vi "Is Last Run.vi"(8 "error in (no error)":errorcluster, 10 "Last Run?":bool, 11 "Model in":refnum<class "Model.lvclass">) -> (0 "error out":errorcluster, 2 "Stop":bool, 3 "Model out":refnum<class "Model.lvclass">)   [LabVIEW 2016, in "Model.lvclass"]
uses:
  Model.lvclass
  Model.lvclass/Model.ctl
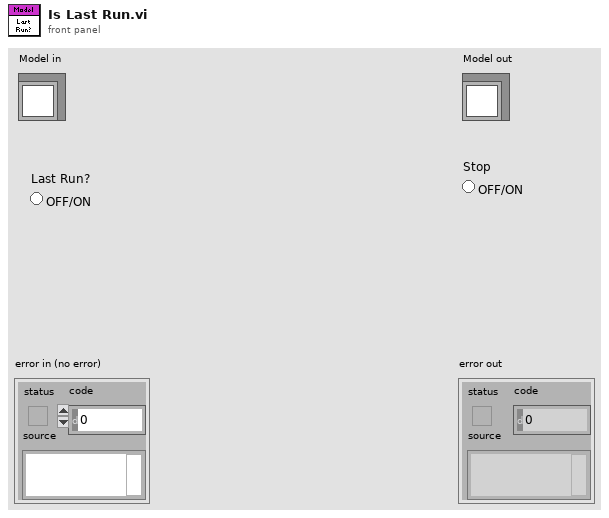
[diagram p1: front panel]
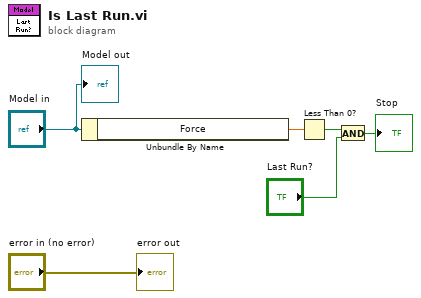
[diagram p0: block diagram]
diagram:
  n1 = Unbundle By Name("Model in") -> ("Force"=w3:dbl)
  n2 = Less Than 0?(x=w3) -> (x < 0?=w2:bool)
  n3 = And(x=w2, y="Last Run?") -> (x .and. y?=→"Stop":bool)
  "error out" <- "error in (no error)"
  "Model out" <- "Model in"
